vi "4. CoffeeMaker Multiple Languages.vi"() -> ()   [LabVIEW 2018]
doc: "Coffee Machine Version 1.0: multiple language support for English, German, and Italian using language data file, and a constant as language selector"
uses:
  Controls/States.ctl
  <vilib>/Utility/file.llb/Read Delimited Spreadsheet (string).vi
panel:
  out "error out":errorcluster
  in  "error in (no error)":errorcluster
  in  "Power Switch":bool caption="Power"
  in  "Simulation":cluster{"Water":dbl, "Coffee":dbl, "Milk":dbl} caption="Wasser" {"Milk" scale=0.0..100.0; "Water" scale=0.0..100.0; "Coffee" scale=0.0..100.0}
  out "Display":T1 {"Coffee" scale=0.0..80.0; "Brewing Chamber" scale=0.0..80.0}
  in  "Coffee Selection":T2 caption="Selezione di Caffè" {"Type" min=0 max=2 scale=0.0..2.0}
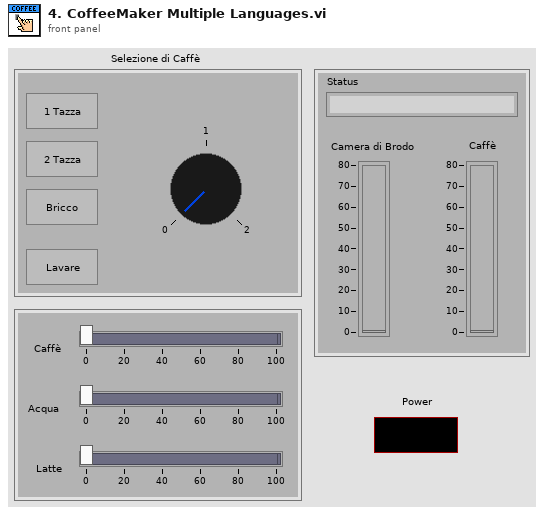
[diagram p1: front panel]
types:
  T1 = cluster{"Brewing Chamber":dbl, "Coffee":dbl, "Status":string}
  T2 = cluster{"1 Cup":bool, "2 Cups":bool, "Pot":bool, "Rinse":bool, "Type":i8}
  T3 = typedef "States.ctl" = enum16{"Initialize", "Set Language", "Wait for Power On", "Heat up", "Check and Wait for Water", "Rinsing", "Check Resources", "User Input", "Grinding", "Boiling", "Pouring", "Rinse before Stop", "Write Data", "Stop"}
  T4 = cluster{"Coffee":refnum<vi>, "Water":refnum<vi>, "Milk":refnum<vi>}
  T5 = cluster{"Status":refnum<vi>, "Brewing Chamber":refnum<vi>, "Coffee":refnum<vi>, "Power Switch":refnum<vi>}
  T6 = cluster{"Coffee Selection":refnum<vi>, "1 Cup":refnum<vi>, "2 Cups":refnum<vi>, "Pot":refnum<vi>, "Rinse":refnum<vi>, "Type":refnum<vi>}
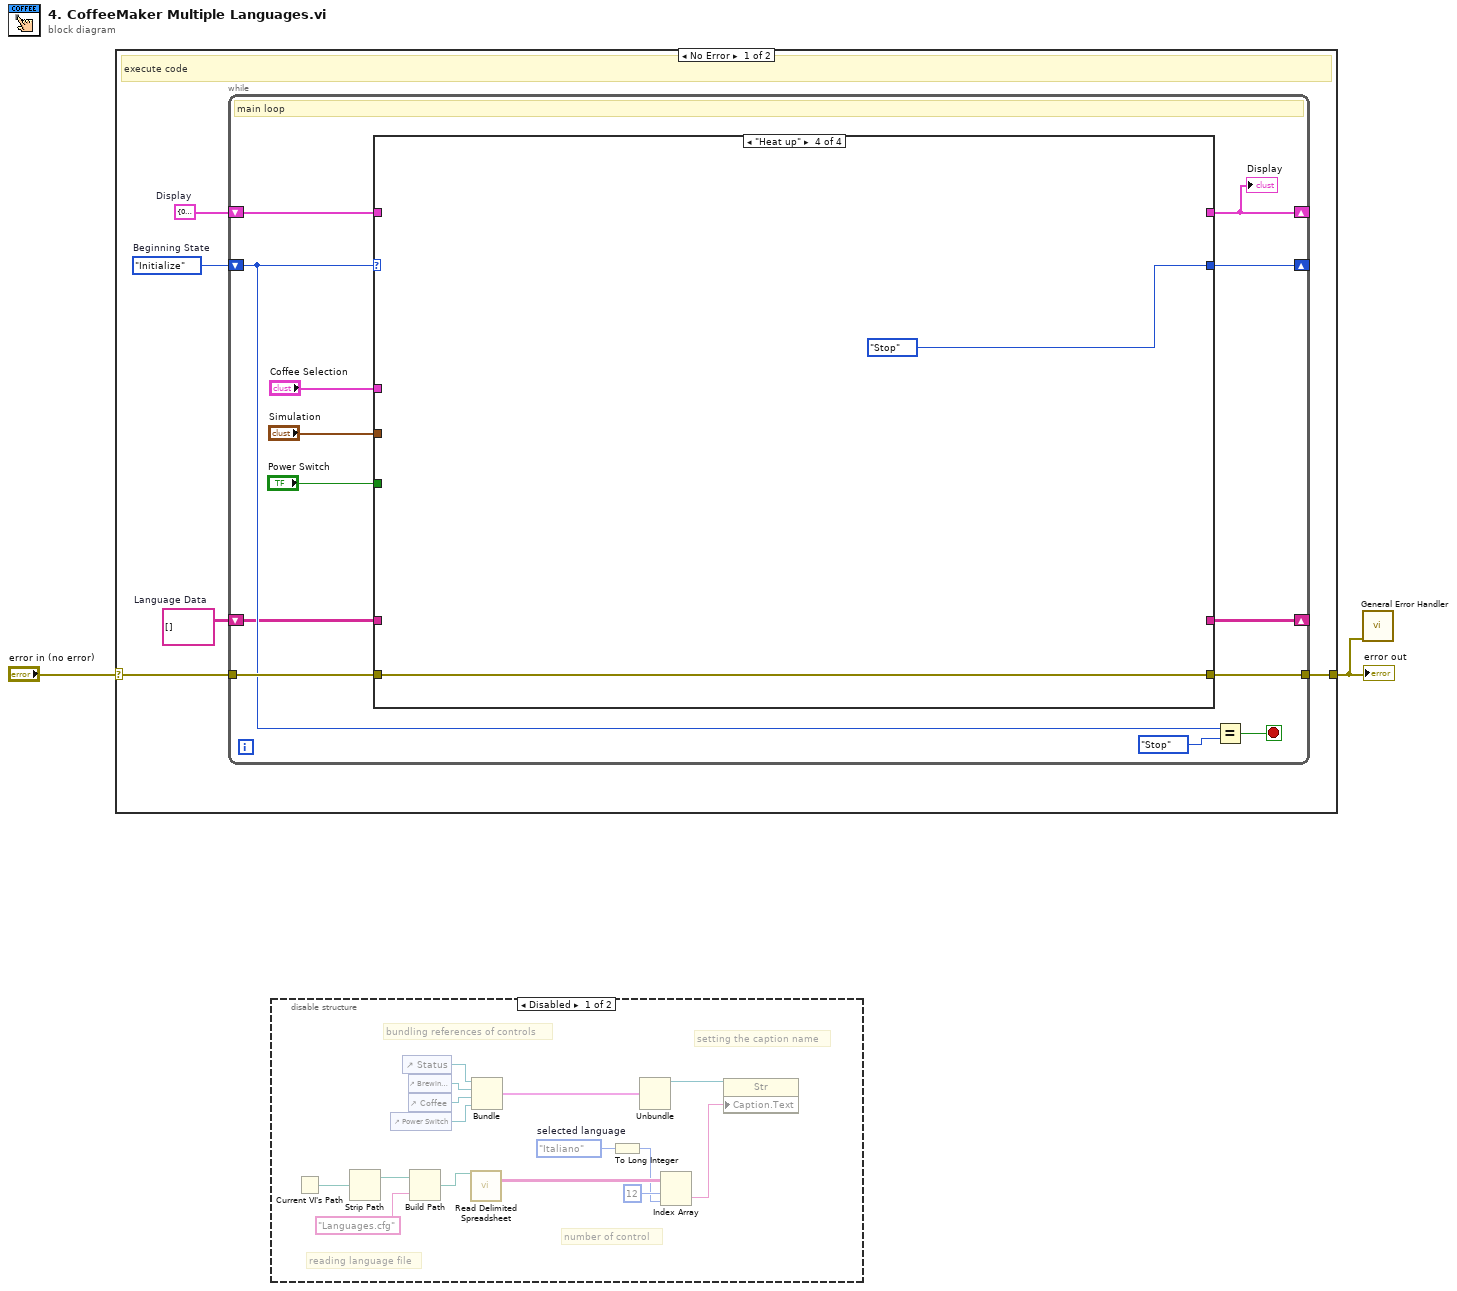
[diagram p0: block diagram]
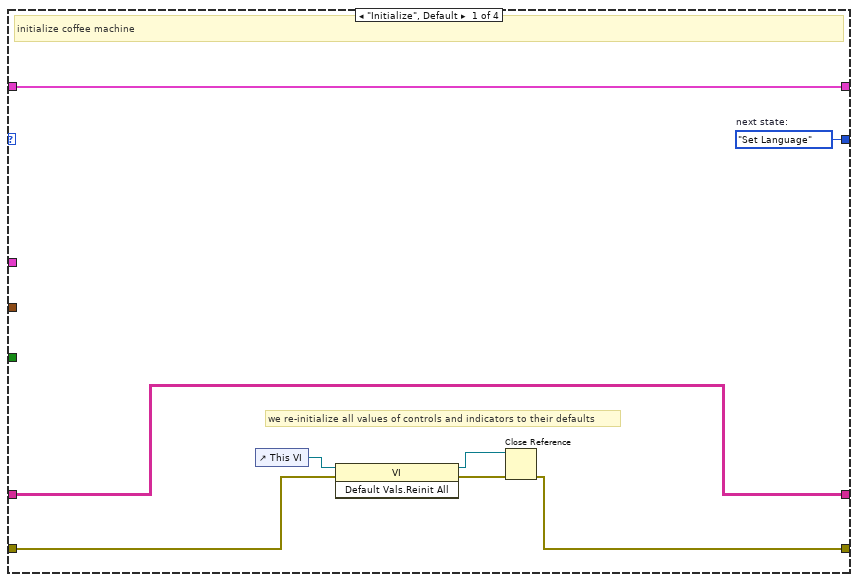
[diagram p3: hidden frame]
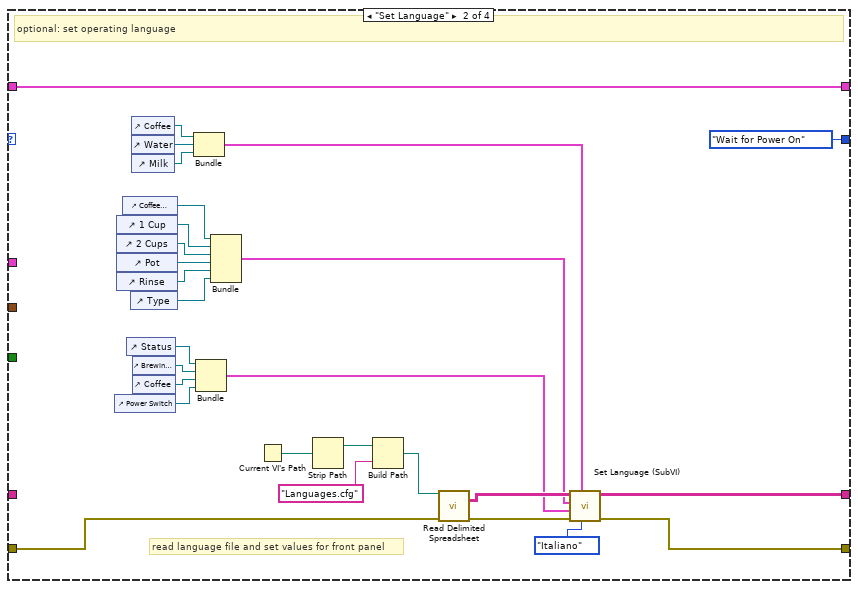
[diagram p4: hidden frame]
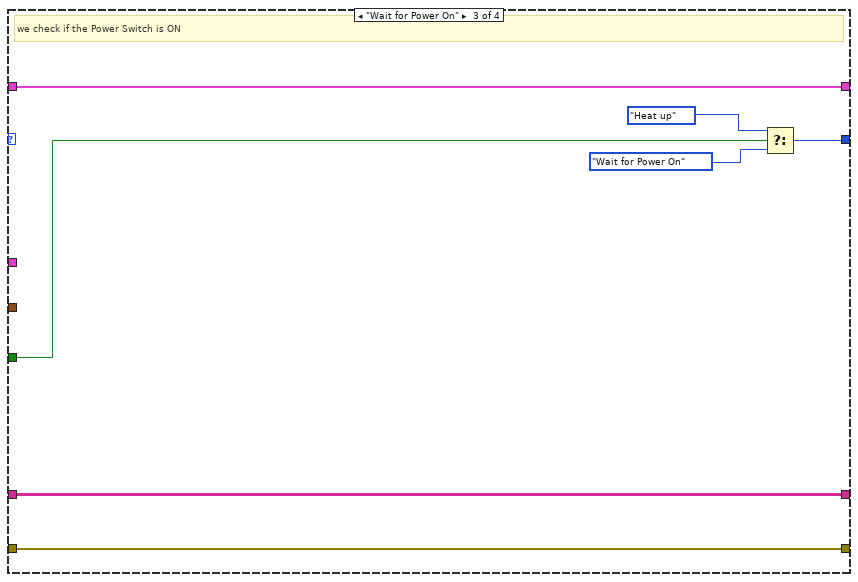
[diagram p5: hidden frame]
diagram:
  n1 = case shown="No Error" "error in (no error)" {
    selector: "error in (no error)" -> [w6 w66]
    tunnel: [w7 w66] -> w1
    frame No Error {
      w3 = string[][] []  # Language Data
      w4 = T1 {"Brewing Chamber"=0.0, "Coffee"=0.0, "Status"=""}  # Display
      w5 = States."Initialize"  # Beginning State
      # "execute code"
      n2 = while {
        tunnel: [w20] -> w7
        tunnel: w6 -> [w19]
        shift-right: [w17] -> _
        shift-left: w5 -> [w16]
        shift-right: [w10] -> _
        shift-left: w3 -> [w8]
        shift-right: [w9] -> _
        shift-left: w4 -> [w13]
        stop <- w14 stop-if-true
        # "main loop"
        n3 = case shown="\"Heat up\"" w16 {
          tunnel: [w22 w49 w59 w65] -> w20
          tunnel: w19 -> [w27 w50 w59 w65]
          tunnel: "Power Switch" -> [_ _ w63 _]
          tunnel: [w24 States."Wait for Power On" ("f") w62 States."Stop" ("f")] -> w17
          tunnel: [w23 w41 w58 _] -> w9
          tunnel: w13 -> [w23 w41 w58 _]
          tunnel: "Coffee Selection" -> [_ _ _ _]
          tunnel: "Simulation" -> [_ _ _ _]
          tunnel: [w21 w48 w57 _] -> w10
          tunnel: w8 -> [w21 _ w57 _]
          frame "Initialize", Default {
            w24 = States."Set Language"  # next state:
            # "we re-initialize all values of controls and indicators to their defaults"
            # "initialize coffee machine"
            n4 = control-ref of="This VI"() -> (w28:refnum<vi>)
            n5 = invoke class="VI" method="Default Vals.Reinit All"(reference=w28, error in=w27) -> (reference out=w26:refnum<vi>, error out=w25:errorcluster)  [unwired: 1 in, 1 out]
            n6 = Close Reference(reference=w26, error in (no error)=w25) -> (error out=w22:errorcluster)
          }
          frame "Set Language" {
            # "read language file and set values for front panel"
            # "optional: set operating language"
            n7 = control-ref of="Power Switch"() -> (w31:refnum<vi>)
            n8 = control-ref of="1 Cup"() -> (w39:refnum<vi>)
            n9 = control-ref of="2 Cups"() -> (w38:refnum<vi>)
            n10 = control-ref of="Pot"() -> (w37:refnum<vi>)
            n11 = control-ref of="Rinse"() -> (w36:refnum<vi>)
            n12 = control-ref of="Coffee Selection"() -> (w40:refnum<vi>)
            n13 = control-ref of="Status"() -> (w34:refnum<vi>)
            n14 = control-ref of="Type"() -> (w35:refnum<vi>)
            n15 = control-ref of="Coffee"() -> (w45:refnum<vi>)
            n16 = control-ref of="Water"() -> (w44:refnum<vi>)
            n17 = control-ref of="Milk"() -> (w43:refnum<vi>)
            n18 = control-ref of="Brewing Chamber"() -> (w33:refnum<vi>)
            n19 = control-ref of="Coffee"() -> (w32:refnum<vi>)
            n20 = Bundle("Coffee"=w45, "Water"=w44, "Milk"=w43) -> (w47:T4)  [unwired: 1 in]
            n21 = Bundle("Status"=w34, "Brewing Chamber"=w33, "Coffee"=w32, "Power Switch"=w31) -> (w29:T5)  [unwired: 1 in]
            n22 = Bundle("Coffee Selection"=w40, "1 Cup"=w39, "2 Cups"=w38, "Pot"=w37, "Rinse"=w36, "Type"=w35) -> (w30:T6)  [unwired: 1 in]
            n23 = Current VI's Path() -> (path=w51:path)
            n24 = Strip Path(path=w51) -> (stripped path=w52:path)  [unwired: 1 out]
            n25 = Build Path(base path=w52, name or relative path="Languages.cfg") -> (appended path=w54:path)
            n26 = call-poly <vilib>:"Read Delimited Spreadsheet.vi"("file path (dialog if empty)"=w54, "error in (no error)"=w50) -> ("all rows"=w56:string[][], "error out"=w55:errorcluster)  [unwired: 8 in, 4 out]
            n27 = call "Set Language (SubVI).vi"("Language (English)"=enum16{"English", "Deutsch", "Italiano"}."Italiano" ("Language"), "Simulation \nReferences"=w47, "error in (no error)"=w55, "Status\nReferences"=w29, "Selection \nReferences"=w30, "Language Data"=w56) -> ("error out"=w49:errorcluster, "Language Data Out"=w48:string[][])  [unwired: 4 in]
          }
          frame "Wait for Power On" {
            # "we check if the Power Switch is ON"
            n28 = Select(t=States."Heat up" ("Beginning State"), s=w63, f=States."Wait for Power On") -> (s? t:f=w62:T3)
          }
          frame "Heat up" {
          }
        }
        "Display" <- w9
        n29 = Equal?(x=w16, y=States."Stop") -> (x = y?=w14:bool)
      }
    }
    frame Error {
      # "do nothing"
    }
  }
  "error out" <- w1
  n30 = disable-structure shown="Disabled" {
    frame Disabled {
      w69 = enum16{"English", "Deutsch", "Italiano"}."Italiano"  # selected language
      # "setting the caption name"
      # "number of control"
      # "reading language file"
      # "bundling references of controls"
      n31 = Current VI's Path() -> (path=w75:path)
      n32 = Strip Path(path=w75) -> (stripped path=w74:path)  [unwired: 1 out]
      n33 = control-ref of="Power Switch"() -> (w81:refnum<vi>)
      n34 = control-ref of="Status"() -> (w78:refnum<vi>)
      n35 = control-ref of="Brewing Chamber"() -> (w79:refnum<vi>)
      n36 = control-ref of="Coffee"() -> (w80:refnum<vi>)
      n37 = Build Path(base path=w74, name or relative path="Languages.cfg") -> (appended path=w72:path)
      n38 = call-poly <vilib>:"Read Delimited Spreadsheet.vi"("file path (dialog if empty)"=w72) -> ("all rows"=w71:string[][])  [unwired: 9 in, 5 out]
      n39 = Bundle("Status"=w78, "Brewing Chamber"=w79, "Coffee"=w80, "Power Switch"=w81) -> (w77:T5)  [unwired: 1 in]
      n40 = To Long Integer(number=w69) -> (32bit integer=w68:i32)
      n41 = Unbundle(w77) -> ("Status"=w76:refnum<vi>)  [unwired: 3 out]
      n42 = Index Array(array=w71, index (row)=12, index (col)=w68) -> (element=w67:string)
      n43 = property class="Str"(reference=w76, "Caption.Text"=w67) -> ()  [unwired: 1 in, 2 out]
    }
    frame Enabled {
    }
  }
  n44 = call <vilib>:"General Error Handler.vi"("error in (no error)"=w1) -> ()  [unwired: 10 in, 5 out]
